vi "Get mode of operation.vi"(7 "timeout (1s)":dbl=1.0 min=0.0, 8 "error in (no error)":errorcluster, 11 "SDO object in":refnum<k20>) -> (0 "error out":errorcluster, 1 "completion code":u32, 3 "SDO object out":refnum<k20>, 6 "Mode of operation":i8(ring) items=["Induction VF – testing purposes only"=-5, "Aligning rotor position"=-4, "Current stepper – testing purposes only "=-3, "Voltage stepper – testing purposes only"=-2, "Voltage constant angle – testing purposes only"=-1, "No mode"=0, "Cyclic sync position"=8, "Cyclic sync velocity"=9, "Cyclic sync torque"=10])   [LabVIEW 2016]
uses:
  <vilib>/CANopenLib/CANOPEN.llb/CANopen SDO Read [I8].vi
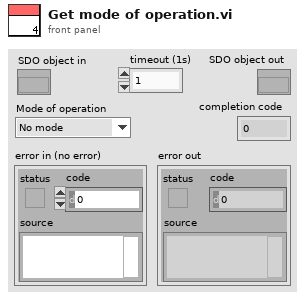
[diagram p1: front panel]
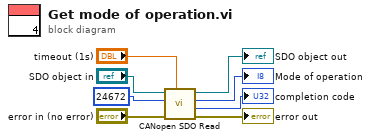
[diagram p0: block diagram]
diagram:
  n1 = call-poly <vilib>:"CANopen SDO Read.vi"("timeout (1s)"="timeout (1s)", "error in (no error)"="error in (no error)", "object index"=u16 24672, "SDO object in"="SDO object in") -> ("error out"=→"error out":errorcluster, "completion code"=→"completion code":u32, "I8 data"=→"Mode of operation":i8, "SDO object out"=→"SDO object out":refnum<k20>)  [unwired: 4 in]
